vi "Library New Path.vi"(4 "error in (no error)":errorcluster, 5 "permissions (system default)":i16=-1, 6 "group (user default)":string, 7 "directory path":path) -> (0 "error out":errorcluster, 3 "dup directory path":path)   [LabVIEW 2012]
doc: "Creates a new directory path. As opposed to the \"New Directory\" function, this VI returns without error if the directory already exists and will first create any as yet non-existent directories leading up to the full directory path."
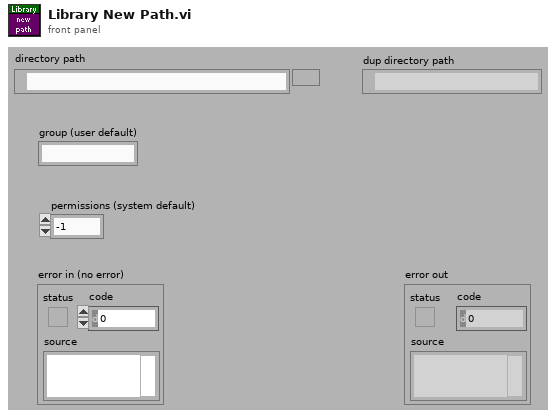
[diagram p1: front panel]
types:
  T1 = typedef "et_Library Error Code Enum.ctl" = enum32{"No error", "Argument error", "Memory is full", "Out of zone", "End of file", "File already open", "Generic file I/O error", "File not found", "File permission error", "Disk is full", "Duplicate path", "Too many files open", "System feature not enabled", "Resource file not found", "Cannot add resource", "Resource not found", "Image not found", "Image memory error", "Pen does not exist", "Config type invalid", "Config token not found", "Config parse error", "Config memory error", "Bad external code format", "Bad external code offset", "External code not present", "Null window", "Destroy window error", "Null menu", "Print aborted", "Bad print record", "Print driver error", "Windows error during printing", "Memory error during printing", "Print dialog error", "Generic print error", "Invalid device refnum", "Device not found", "Device parameter error", "Device unit error", "Cannot open device", "Device call aborted", "Generic error", "Cancelled by user", "Object ID too low", "Object ID too high", "Object not in heap", "Unknown heap", "Unknown object (invalid DefProc)", "Unknown object (DefProc not in table)", "Message out of range", "Invalid (null) method", "Unknown message", "Manager call not supported", "Bad address", "Network operation in progress", "Network operation timed out", "Connection is busy", "Network attribute not supported", "Network error", "Address in use", "System out of memory", "Connection aborted", "Connection refused", "Not connected", "Already connected", "Connection closed", "Initialization error (interapplication manager)", "Bad occurrence", "Wait on unbound occurrence handler", "Occurrence queue overflow", "Datalog type conflict", "Unused", "Unrecognized type (interapplication manager)", "Memory corrupt", "Failed to make temporary DLL", "Old CIN version", "Drag socket not found", "Failed to load drop-object", "Failed to register OLE object", "Failed to release OLE object", "Format specifier type mismatch", "Unknown format specifier", "Too few format specifiers", "Too many format specifiers", "Scan failed", "Newer CIN version", "Error converting to variant", "Runtime menu error", "Password tampered", "Variant attribute not found", "Incompatible variant data type", "Event data is not available", "Event Store is not present", "Occurrence is not found", "Event Queue is not created", "Event info is not available in the type library", "Refnum passed is NULL", "Error retrieving Class GUID", "Error retrieving CoClass GUID", "Error retrieving TypeLib GUID.", "Bad built application magic bytes.", "Specific driver is different from the specific driver associated with the Logical Name.", "There is no session opened to the class driver.", "Max Error", "MAX - Error with config objects", "MAX - Error loading configuration", "MAX - Group not supported", "Singlecast connections can not send to multicast addresses.", "Multicast connections can not send to singlecast addresses.", "Specified IP address not in multicast address range.", "Attempt to write to read-only multicast connection.", "Attempt to read from write-only multicast connection.", "The buffer used to receive a datagram was smaller than the datagram itself", "Error code not enumerated"}
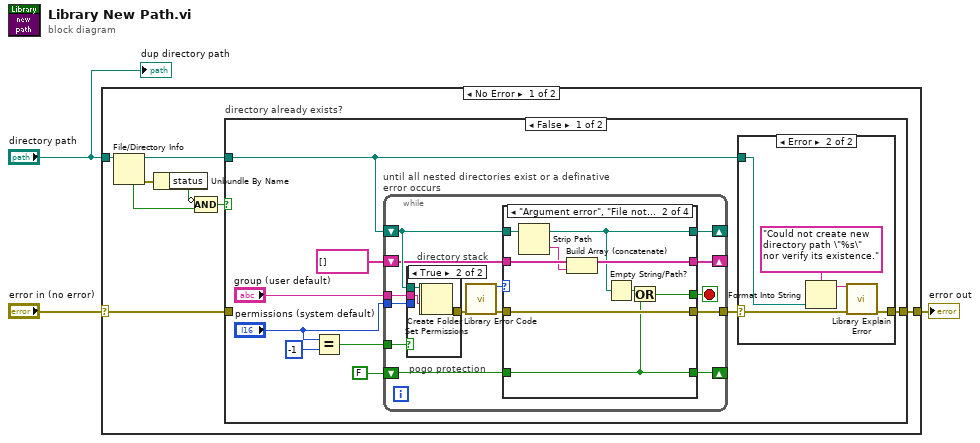
[diagram p0: block diagram]
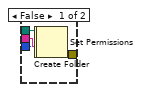
[diagram p3: hidden frame]
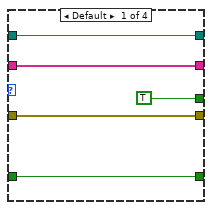
[diagram p4: hidden frame]
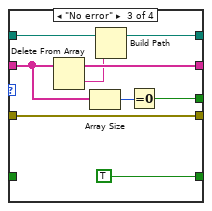
[diagram p5: hidden frame]
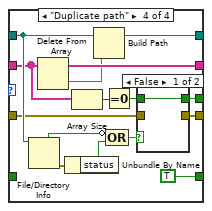
[diagram p6: hidden frame]
diagram:
  n1 = case shown="No Error" "error in (no error)" {
    selector: "error in (no error)" -> [w4 w94]
    tunnel: [w11 w94] -> w3
    tunnel: "directory path" -> [w10 _]
    frame No Error {
      n2 = File/Directory Info(path=w10) -> (path out=w7:path, directory=w5:bool, error out=w9:errorcluster)  [unwired: 1 in, 4 out]
      n3 = Unbundle By Name(w9) -> ("status"=w6:bool)
      n4 = Compound Arithmetic op=AND(invert w6, w5) -> (w8:bool)
      n5 = case "directory already exists?" shown="False" w8 {
        tunnel: [w18 w93] -> w11
        tunnel: w7 -> [w16 _]
        tunnel: w4 -> [_ w93]
        frame False {
          n6 = Equal?(x="permissions (system default)", y=i16 -1) -> (x = y?=w12:bool)
          n7 = while "until all nested directories exist or a definative error occurs" {
            shift-right: [w35] -> _
            shift-left: w16 -> [w36]
            tunnel: [w37] -> w15
            shift-right: [w34] -> _
            shift-left: string[] [] -> [w33]
            shift-right: [w30] -> _
            shift-left: FALSE -> [w31]
            tunnel: "group (user default)" -> [w29]
            tunnel: "permissions (system default)" -> [w28]
            tunnel: w12 -> [w27]
            stop <- w32 stop-if-true
            # "directory stack"
            # "pogo protection"
            n8 = case shown="True" w27 {
              tunnel: [w46 w51] -> w40
              tunnel: w36 -> [w45 w50]
              tunnel: w29 -> [w44 w49]
              tunnel: w28 -> [w43 _]
              frame False {
                n9 = Create Folder(path (use dialog)=w45) -> (created path=w42:path, error out=w41:errorcluster)  [unwired: 2 in, 1 out]
                n10 = Set Permissions(7:w43, 8:w41, 9:w44, 11:w42) -> (0:w46:errorcluster)  [unwired: 1 in, 1 out]
              }
              frame True {
                n11 = Create Folder(path (use dialog)=w50) -> (created path=w48:path, error out=w47:errorcluster)  [unwired: 2 in, 1 out]
                n12 = Set Permissions(8:w47, 9:w49, 11:w48) -> (0:w51:errorcluster)  [unwired: 2 in, 1 out]
              }
            }
            n13 = call "Library Error Code.vi"("error"=w40) -> ("error code enum"=w39:T1, "dup error"=w38:errorcluster)  [unwired: 12 in, 1 out]
            n14 = case shown="\"Argument error\", \"File not found\"" w39 {
              tunnel: w38 -> [w56 w61 w68 w79]
              tunnel: [w56 w61 w68 w78] -> w37
              tunnel: w36 -> [w55 w65 w74 w85]
              tunnel: [w55 w59 w71 w88] -> w35
              tunnel: [w54 w63 w73 w89] -> w34
              tunnel: w33 -> [w54 w64 w66 w75]
              tunnel: [TRUE w58 w72 w80] -> w32
              tunnel: w31 -> [w52 w57 _ _]
              tunnel: [w52 w57 TRUE TRUE] -> w30
              frame Default {
              }
              frame "Argument error", "File not found" {
                n15 = Strip Path(path=w65) -> (stripped path=w59:path, name=w62:string)
                n16 = Build Array (concatenate)(w64, w62) -> (w63:string[])
                n17 = Empty String/Path?(string/path=w59) -> (empty?=w60:bool)
                n18 = Or(x=w60, y=w57) -> (x .or. y?=w58:bool)
              }
              frame "No error" {
                n19 = Delete From Array(array=w66) -> (deleted portion=w70:string, array with subset deleted=w73:string[])  [unwired: 2 in]
                n20 = Array Size(array=w66) -> (size(s)=w67:i32)
                n21 = Build Path(base path=w74, name or relative path=w70) -> (appended path=w71:path)
                n22 = Equal To 0?(x=w67) -> (x = 0?=w72:bool)
              }
              frame "Duplicate path" {
                n23 = File/Directory Info(path=w85) -> (directory=w82:bool, error out=w84:errorcluster)  [unwired: 1 in, 5 out]
                n24 = Delete From Array(array=w75) -> (deleted portion=w87:string, array with subset deleted=w89:string[])  [unwired: 2 in]
                n25 = Unbundle By Name(w84) -> ("status"=w83:bool)
                n26 = Array Size(array=w75) -> (size(s)=w76:i32)
                n27 = Build Path(base path=w85, name or relative path=w87) -> (appended path=w88:path)
                n28 = Equal To 0?(x=w76) -> (x = 0?=w77:bool)
                n29 = Compound Arithmetic op=OR(invert w82, w83) -> (w81:bool)
                n30 = case shown="False" w81 {
                  selector: w81 -> [_ w91]
                  tunnel: w77 -> [w90 _]
                  tunnel: [w90 w91] -> w80
                  tunnel: w79 -> [_ w92]
                  tunnel: [_ w92] -> w78
                  frame False {
                  }
                  frame True {
                  }
                }
              }
            }
          }
          n31 = case shown="Error" w15 {
            selector: w15 -> [w21 w23]
            tunnel: [w21 w26] -> w18
            tunnel: w16 -> [_ w22]
            frame No Error {
            }
            frame Error {
              n32 = Format Into String(format string="Could not create new directory path \"%s\" nor verify its existence.", w22) -> (resulting string=w24:string)  [unwired: 2 in, 1 out]
              n33 = call "Library Explain Error.vi"("explanation prefix (none)"=w24, "error in (no error)"=w23) -> ("explained error"=w26:errorcluster)  [unwired: 13 in]
            }
          }
        }
        frame True {
        }
      }
    }
    frame Error {
    }
  }
  "error out" <- w3
  "dup directory path" <- "directory path"
